vi "Initialize.vi"(8 "error in (no error)":errorcluster, 11 "ATS9462 Class in":refnum<class "ATS9462 Class.lvclass">) -> (0 "error out":errorcluster, 3 "ATS9462 Class out":refnum<class "ATS9462 Class.lvclass">)   [LabVIEW 2014, in "ATS9462 Class.lvclass"]
uses:
  ATS9462 Class.lvclass
  ATS-VI/ATS_ctl/Device_Ctrl.ctl
  ATS-VI/ATS_ctl/ATS_Check_Ctrl.ctl
  DAQ Parameters.ctl
  Trigger Source.ctl
  Trigger Slope.ctl
  Type Defs/OCT DAQ Channel Data Type.ctl
  Clock Control.ctl
  DAQ Class.lvclass
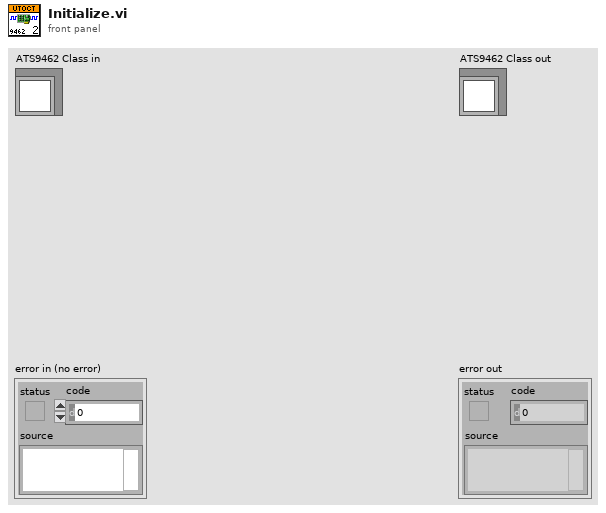
[diagram p1: front panel]
types:
  T1 = typedef "DAQ Class.lvclass/DAQ Parameters.ctl" = cluster{"Points Per A-Scan":u32, "A-Scans Per B-Scan":u32, "Number of B-Scans":u32, "A-Scans Per Transfer":u32, "Trigger Voltage":sgl, "Trigger Source":T2, "Trigger Slope":T3, "Channel":T4, "Clock":T5, "Bits per Sample":dbl, "Range":dbl}
  T2 = typedef "DAQ Class.lvclass/Trigger Source.ctl" = enum16{"External", "Channel A", "Channel B"}
  T3 = typedef "DAQ Class.lvclass/Trigger Slope.ctl" = enum16{"Rising", "Falling"}
  T4 = typedef "OCT DAQ Channel Data Type.ctl" = enum16{"Channel 1", "Channel 2", "Channel 1 and 2"}
  T5 = typedef "DAQ Class.lvclass/Clock Control.ctl" = enum16{"Internal Clock", "External Clock"}
  T6 = typedef "ATS_Check_Ctrl.ctl" = enum16{"None", "NO_ATS9462", "ATS9462_Traditional", "Verify Board", "OnBoard Memory", "Board & Memory", "Master/Slave", "NO Master/Slave"}
  T7 = typedef "Device_Ctrl.ctl" = enum16{"Status", "About", "Arm", "ForceTrig", "Abort", "Initialize", "Init (NoPreset)", "Info", "Close", "Calibrate", "SetManually", "LED_ON", "LED_OFF"}
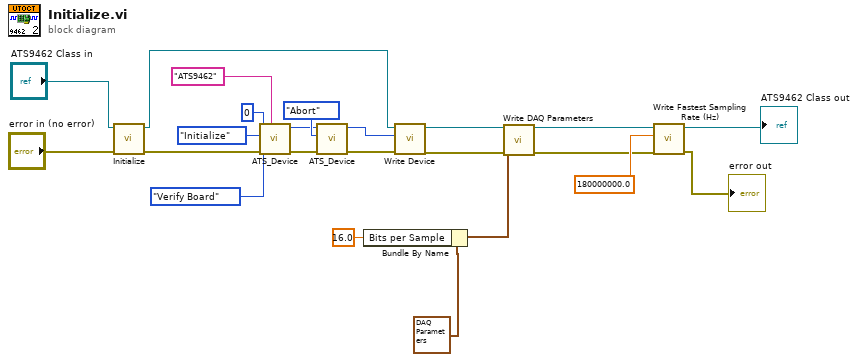
[diagram p0: block diagram]
diagram:
  n1 = call-parent "Initialize.vi"("error in (no error)"="error in (no error)", "DAQ Class in"="ATS9462 Class in") -> ("error out"=w15:errorcluster, "DAQ Class out"=w12:refnum<class "ATS9462 Class.lvclass">)  [unwired: 8 in]
  n2 = call "ATS_Device.vi"("BoardToVerify"="ATS9462", "error in (no error)"=w15, "ATS_Check"=ATS_Check_Ctrl."Verify Board", "DevCtrl"=Device_Ctrl."Initialize", "DeviceIn"=0 ("Device")) -> ("error out"=w16:errorcluster, "DeviceOut"=w19:i32)  [unwired: 5 out]
  n3 = call "ATS_Device.vi"("error in (no error)"=w16, "DevCtrl"=Device_Ctrl."Abort", "DeviceIn"=w19) -> ("error out"=w14:errorcluster, "DeviceOut"=w13:i32)  [unwired: 2 in, 5 out]
  n4 = Bundle By Name(cluster=T1 {"Points Per A-Scan"=0, "A-Scans Per B-Scan"=0, "Number of B-Scans"=0, "A-Scans Per Transfer"=0, "Trigger Voltage"=0.0, "Trigger Source"=enum."External", "Trigger Slope"=enum."Rising", "Channel"=enum."Channel 1", "Clock"=enum."Internal Clock", "Bits per Sample"=0.0, "Range"=0.0} ("DAQ Parameters"), "Bits per Sample"=16.0) -> (w7:T1)
  n5 = call-dynamic "Write Device.vi"("error in (no error)"=w14, "Device"=w13, "ATS9462 Class in"=w12) -> ("error out"=w3:errorcluster, "ATS9462 Class out"=w4:refnum<class "ATS9462 Class.lvclass">)  [unwired: 7 in]
  n6 = call-dynamic "Write DAQ Parameters.vi"("error in (no error)"=w3, "DAQ Parameters"=w7, "ATS9462 Class in"=w4) -> ("error out"=w2:errorcluster, "ATS9462 Class out"=w1:refnum<class "ATS9462 Class.lvclass">)  [unwired: 7 in]
  n7 = call-dynamic "Write Fastest Sampling Rate (Hz).vi"("error in (no error)"=w2, "Fastest Sampling Rate (Hz)"=180000000.0, "DAQ Class in"=w1) -> ("error out"=→"error out":errorcluster, "DAQ Class out"=→"ATS9462 Class out":refnum<class "ATS9462 Class.lvclass">)  [unwired: 7 in]
